vi "WalkDownTree.vi"(8 "error in":errorcluster, 10 "Node In":variant, 11 "Qualified Name":string) -> (0 "error out":errorcluster, 2 "Nodes Out":variant[](array[variant]), 3 "Names":string[](array[string]))   [LabVIEW 2019, in "Tree.lvclass"]
uses:
  Tree.lvclass
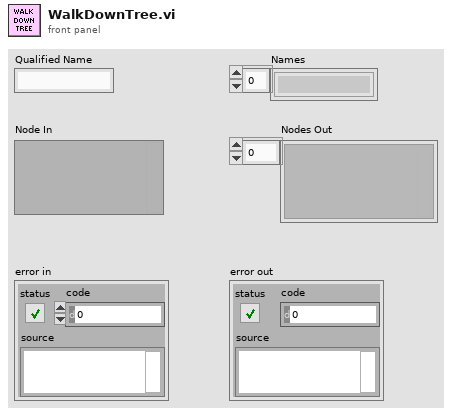
[diagram p1: front panel]
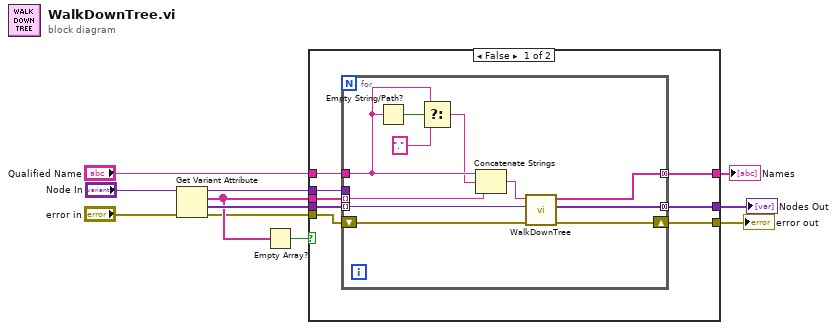
[diagram p0: block diagram]
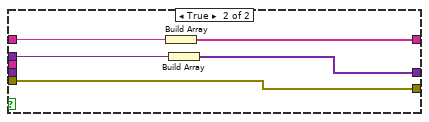
[diagram p2: hidden frame]
diagram:
  n1 = Get Variant Attribute(Variant="Node In", error in="error in") -> (duplicate Variant=w11:variant, names=w8:string[], values=w10:variant[], error out=w2:errorcluster)  [unwired: 2 in]
  n2 = Empty Array?(array=w8) -> (empty?=w7:bool)
  n3 = case shown="False" w7 {
    tunnel: w11 -> [w19 w33]
    tunnel: w10 -> [w18 _]
    tunnel: w8 -> [w17 _]
    tunnel: "Qualified Name" -> [w16 w35]
    tunnel: [w14 w34] -> w5
    tunnel: [w15 w32] -> w4
    tunnel: w2 -> [w13 w31]
    tunnel: [w12 w31] -> w1
    frame False {
      n4 = for {
        tunnel: w19 -> [_]
        tunnel: w17 -> [w28] mode=indexing
        tunnel: w18 -> [w30] mode=indexing
        tunnel: w16 -> [w22]
        tunnel: [w27] -> w15 mode=concatenating
        tunnel: [w26] -> w14 mode=concatenating
        shift-right: [w25] -> w12
        shift-left: w13 -> [w24]
        n5 = Empty String/Path?(string/path=w22) -> (empty?=w23:bool)
        n6 = Select(t=w22, s=w23, f="." ("string")) -> (s? t:f=w20:string)
        n7 = Concatenate Strings(w22, w20, w28) -> (w29:string)
        n8 = call "WalkDownTree.vi"("error in"=w24, "Node In"=w30, "Qualified Name"=w29) -> ("error out"=w25:errorcluster, "Nodes Out"=w27:variant[], "Names"=w26:string[])  [unwired: 6 in]
      }
    }
    frame True {
      n9 = Build Array(w35) -> (w34:string[])
      n10 = Build Array(w33) -> (w32:variant[])
    }
  }
  "Nodes Out" <- w4
  "Names" <- w5
  "error out" <- w1
